vi "GET_Running_perc._and_travel_(online).vi"(8 "Reset? (F)":bool, 9 "Animal coordinates in":T1, 10 "Histogram parameters":T3, 11 "Running stats results in":T2) -> (3 "Running stats results out":T2)   [LabVIEW 2018, in "Tracker.lvlib"]
uses:
  Tracker.lvlib
  Controls/CTL_Histogram_parameters.ctl
  Controls/CTL_Running_statistics_results.ctl
  Controls/CTL_Animal_Coordinates_and_Speed.ctl
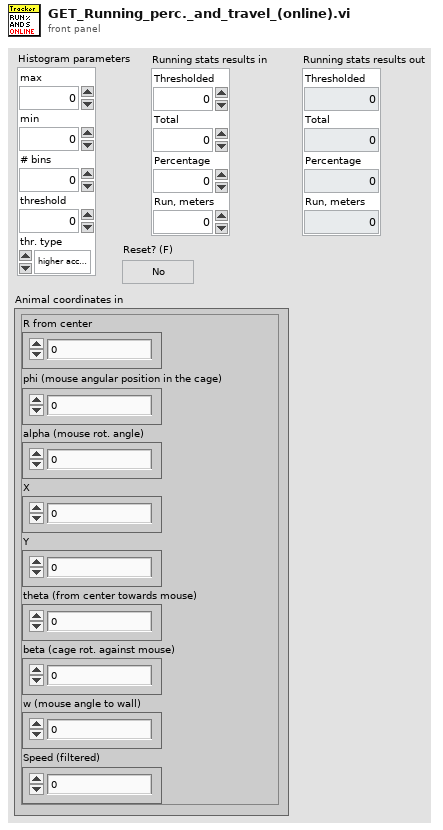
[diagram p1: front panel]
types:
  T1 = typedef "Tracker.lvlib/CTL_Animal_Coordinates_and_Speed.ctl" = cluster{"R from center":dbl, "phi (mouse angular position in the cage)":dbl, "alpha (mouse rot. angle)":dbl, "X":dbl, "Y":dbl, "theta (from center towards mouse)":dbl, "beta (cage rot. against mouse)":dbl, "w (mouse angle to wall)":dbl, "Speed (filtered)":dbl}
  T2 = typedef "CTL_Running_statistics_results.ctl" = cluster{"Thresholded":u32, "Total":u32, "Percentage":dbl, "Run, meters":dbl}
  T3 = typedef "Tracker.lvlib/CTL_Histogram_parameters.ctl" = cluster{"max":dbl, "min":dbl, "# bins":i32, "threshold":dbl, "thr. type":enum16{"higher accepted", "lower accepted"}}
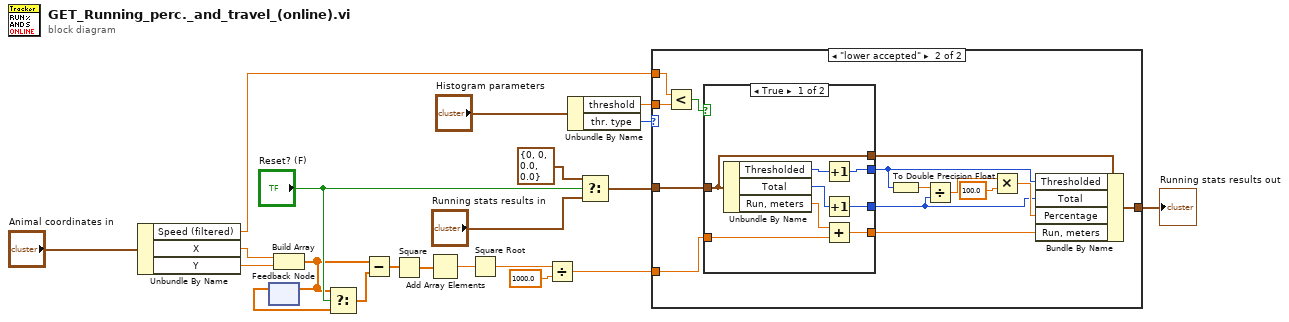
[diagram p0: block diagram]
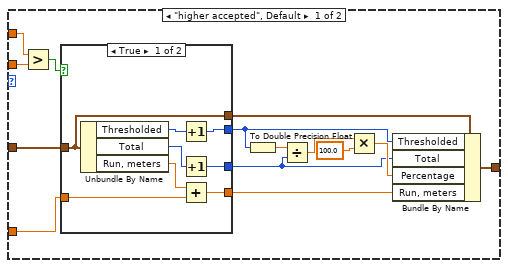
[diagram p2: hidden frame]
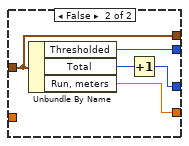
[diagram p3: hidden frame]
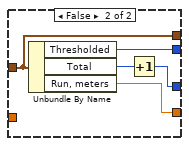
[diagram p4: hidden frame]
diagram:
  n1 = Unbundle By Name("Animal coordinates in") -> ("Speed (filtered)"=w15:dbl, "X"=w14:dbl, "Y"=w13:dbl)
  n2 = feedback #1() -> (w12:dbl[])  [unwired: 1 in]
  n3 = Build Array(w14, w13) -> (w6:dbl[])
  n4 = feedback-in #1(w6) -> ()
  n5 = Select(t=w6, s="Reset? (F)", f=w12) -> (s? t:f=w8:dbl[])
  n6 = Subtract(x=w6, y=w8) -> (x-y=w11:dbl[])
  n7 = Square(x=w11) -> (x^2=w10:dbl[])
  n8 = Add Array Elements(numeric array=w10) -> (sum=w9:dbl)
  n9 = Square Root(x=w9) -> (sqrt(x)=w4:dbl)
  n10 = Divide(x=w4, y=1000.0) -> (x/y=w1:dbl)
  n11 = Unbundle By Name("Histogram parameters") -> ("threshold"=w19:dbl, "thr. type"=w20:enum16{"higher accepted", "lower accepted"})
  n12 = Select(t=T2 {"Thresholded"=0, "Total"=0, "Percentage"=0.0, "Run, meters"=0.0} ("Running stats results"), s="Reset? (F)", f="Running stats results in") -> (s? t:f=w18:T2)
  n13 = case shown="\"lower accepted\"" w20 {
    tunnel: w15 -> [w35 w62]
    tunnel: w19 -> [w34 w61]
    tunnel: w18 -> [w24 w51]
    tunnel: [w25 w52] -> w2
    tunnel: w1 -> [w22 w49]
    frame "higher accepted", Default {
      n14 = Greater?(x=w35, y=w34) -> (0:w33:bool)
      n15 = case shown="True" w33 {
        tunnel: w24 -> [w39 w45]
        tunnel: [w41 w47] -> w27
        tunnel: [w40 w46] -> w26
        tunnel: [w39 w45] -> w29
        tunnel: [w36 w44] -> w23
        tunnel: w22 -> [w38 _]
        frame True {
          n16 = Unbundle By Name(w39) -> ("Thresholded"=w43:u32, "Total"=w42:u32, "Run, meters"=w37:dbl)
          n17 = Increment(x=w43) -> (x+1=w40:u32)
          n18 = Increment(x=w42) -> (x+1=w41:u32)
          n19 = Add(x=w37, y=w38) -> (x+y=w36:dbl)
        }
        frame False {
          n20 = Unbundle By Name(w45) -> ("Thresholded"=w46:u32, "Total"=w48:u32, "Run, meters"=w44:dbl)
          n21 = Increment(x=w48) -> (x+1=w47:u32)
        }
      }
      n22 = To Double Precision Float(number=w26) -> (double precision float=w32:dbl)
      n23 = Divide(x=w32, y=w27) -> (x/y=w31:dbl)
      n24 = Multiply(x=w31, y=100.0) -> (x*y=w28:dbl)
      n25 = Bundle By Name(cluster=w29, "Thresholded"=w26, "Total"=w27, "Percentage"=w28, "Run, meters"=w23) -> (w25:T2)
    }
    frame "lower accepted" {
      n26 = Less?(x=w62, y=w61) -> (x < y?=w60:bool)
      n27 = case shown="True" w60 {
        tunnel: w51 -> [w66 w72]
        tunnel: [w68 w74] -> w54
        tunnel: [w67 w73] -> w53
        tunnel: [w66 w72] -> w56
        tunnel: [w63 w71] -> w50
        tunnel: w49 -> [w65 _]
        frame True {
          n28 = Unbundle By Name(w66) -> ("Thresholded"=w70:u32, "Total"=w69:u32, "Run, meters"=w64:dbl)
          n29 = Increment(x=w70) -> (x+1=w67:u32)
          n30 = Increment(x=w69) -> (x+1=w68:u32)
          n31 = Add(x=w64, y=w65) -> (x+y=w63:dbl)
        }
        frame False {
          n32 = Unbundle By Name(w72) -> ("Thresholded"=w73:u32, "Total"=w75:u32, "Run, meters"=w71:dbl)
          n33 = Increment(x=w75) -> (x+1=w74:u32)
        }
      }
      n34 = To Double Precision Float(number=w53) -> (double precision float=w59:dbl)
      n35 = Divide(x=w59, y=w54) -> (x/y=w58:dbl)
      n36 = Multiply(x=w58, y=100.0) -> (x*y=w55:dbl)
      n37 = Bundle By Name(cluster=w56, "Thresholded"=w53, "Total"=w54, "Percentage"=w55, "Run, meters"=w50) -> (w52:T2)
    }
  }
  "Running stats results out" <- w2
